vi "读取信号灯.vi"(8 "error in (no error)":errorcluster caption="错误输入（无错误）", 11 "信号灯成员类.lvclass输入":refnum<class "信号灯成员类.lvclass">) -> (0 "error out":errorcluster caption="错误输出", 2 "信号灯":bool[](array[boolean]), 3 "信号灯成员类.lvclass输出":refnum<class "信号灯成员类.lvclass">)   [LabVIEW 2017, in "信号灯成员类.lvclass"]
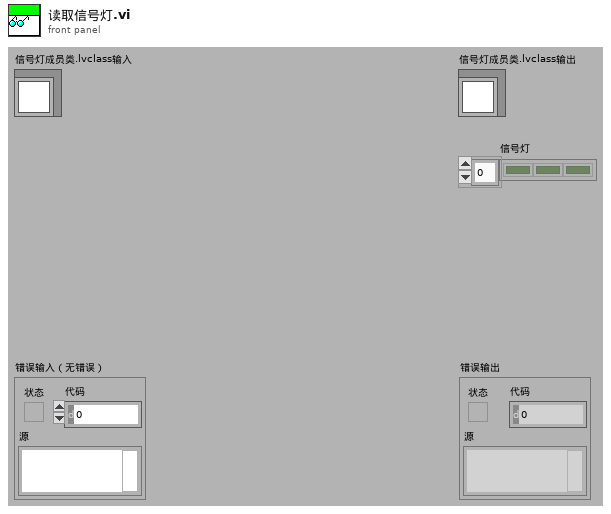
[diagram p1: front panel]
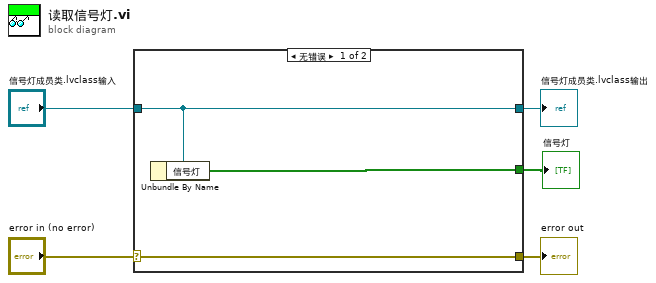
[diagram p0: block diagram]
diagram:
  n1 = case shown="无错误" "error in (no error)" {
    selector: "error in (no error)" -> [w8 w9]
    tunnel: [w8 w9] -> w4
    tunnel: [w7 w10] -> w2
    tunnel: "信号灯成员类.lvclass输入" -> [w7 w10]
    tunnel: [w6 _] -> w1
    frame No Error {
      n2 = Unbundle By Name(w7) -> ("信号灯"=w6:bool[])
    }
    frame Error {
    }
  }
  "error out" <- w4
  "信号灯成员类.lvclass输出" <- w2
  "信号灯" <- w1
